vi "Heat2D_Solve X Direction.vi"(4 "F(t, x, y)":dbl[][][](array[numeric]), 5 "Coefficients":T2, 6 "step":i32, 7 "TriDia Cluster":T1, 8 "Boundary Condition":cluster{"type":T3, "Value":dbl[][]}[](array[cluster]) {"type" items=["Dirichlet", "Neumann"]}, 9 "U(n)":dbl[][](array[numeric]), 10 "Matr_RHS":dbl[][](array[numeric]), 11 "X RHS":dbl[][](array[numeric])) -> (1 "U(n+1/2)":dbl[][](array[numeric]), 3 "X RHS out":dbl[][](array[numeric]))   [LabVIEW 2020, in "NI_PDE.lvlib"]
uses:
  <vilib>/gmath/NI_PDE.lvlib
  <vilib>/gmath/pde.llb/Common/PDE_BC Type.ctl
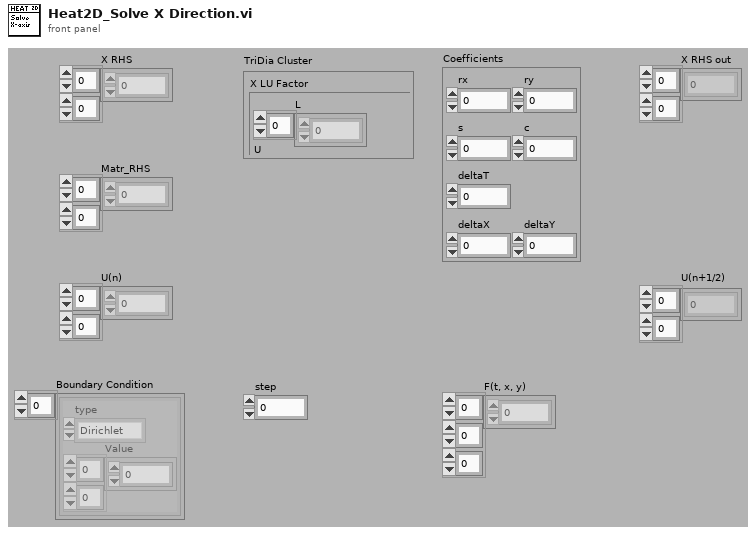
[diagram p1: front panel]
types:
  T1 = cluster{"X LU Factor":cluster{"L":dbl[], "U":cluster{"Diagonal":dbl[], "Super Diagonal":dbl[], "2nd Super Diagonal":dbl[]}, "Pivot":i32[]}, "Y LU Factor":cluster{"L":dbl[], "U":cluster{"Diagonal":dbl[], "Super Diagonal":dbl[], "2nd Super Diagonal":dbl[]}, "Pivot":i32[]}, "X Tridiagonal":cluster{"SubDiagonal":dbl[], "MainDiagonal":dbl[], "SuperDiagonal":dbl[]}, "Y Tridiagonal":cluster{"SubDiagonal":dbl[], "MainDiagonal":dbl[], "SuperDiagonal":dbl[]}}
  T2 = cluster{"rx":dbl, "ry":dbl, "s":dbl, "c":dbl, "deltaT":dbl, "deltaX":dbl, "deltaY":dbl}
  T3 = typedef "NI_PDE.lvlib/PDE_BC Type.ctl" = i32
  T4 = cluster{"L":dbl[], "U":cluster{"Diagonal":dbl[], "Super Diagonal":dbl[], "2nd Super Diagonal":dbl[]}, "Pivot":i32[]}
  T5 = cluster{"SubDiagonal":dbl[], "MainDiagonal":dbl[], "SuperDiagonal":dbl[]}
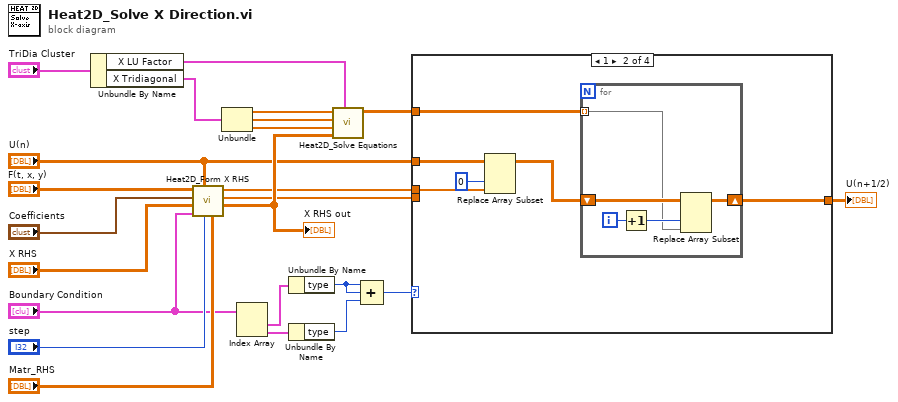
[diagram p0: block diagram]
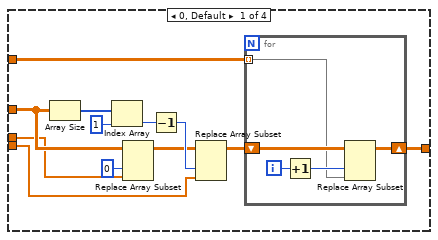
[diagram p2: hidden frame]
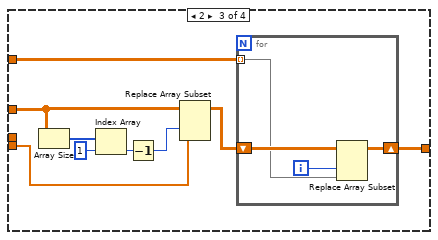
[diagram p3: hidden frame]
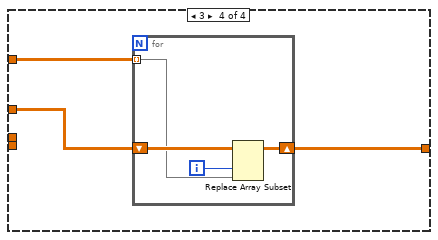
[diagram p4: hidden frame]
diagram:
  n1 = Unbundle By Name("TriDia Cluster") -> ("X LU Factor"=w10:T4, "X Tridiagonal"=w9:T5)
  n2 = call <vilib>:"Heat2D_Form X RHS.vi"("Matr_RHS"="Matr_RHS", "step"="step", "U(n)"="U(n)", "Boundary Condition"="Boundary Condition", "X RHS"="X RHS", "Coefficients"="Coefficients", "F(t, x, y)"="F(t, x, y)") -> ("X RHS out"=w13:dbl[][], "U(M)"=w1:dbl[], "U(0)"=w4:dbl[])  [unwired: 2 out]
  "X RHS out" <- w13
  n3 = Unbundle(w9) -> ("SubDiagonal"=w16:dbl[], "MainDiagonal"=w15:dbl[], "SuperDiagonal"=w14:dbl[])
  n4 = Index Array(array="Boundary Condition") -> (element #1=w20:cluster{"type":T3, "Value":dbl[][]}, element #2=w19:cluster{"type":T3, "Value":dbl[][]})  [unwired: 2 in]
  n5 = Unbundle By Name(w20) -> ("type"=w18:T3)
  n6 = Unbundle By Name(w19) -> ("type"=w17:T3)
  n7 = call <vilib>:"Heat2D_Solve Equations.vi"("LU Factor"=w10, "RHS"=w13, "SuperDiagonal"=w14, "MainDiagonal"=w15, "SubDiagonal"=w16) -> ("Solution Vector"=w6:dbl[][])  [unwired: 6 out]
  n8 = Compound Arithmetic op=ADD(w18, w18, w17) -> (w3:T3)
  n9 = case shown="1" w3 {
    tunnel: w6 -> [w26 w43 w53 w66]
    tunnel: [w25 w41 w52 w65] -> w2
    tunnel: w4 -> [w28 w45 _ _]
    tunnel: w1 -> [w24 _ w55 _]
    tunnel: "U(n)" -> [w29 w46 w56 w67]
    frame 0, Default {
      n10 = Array Size(array=w29) -> (size(s)=w31:i32[])
      n11 = Index Array(array=w31, index=1) -> (element=w32:i32)
      n12 = Replace Array Subset(array=w29, new element=w28, index (col)=0 ("index (row)")) -> (w30:dbl[][])  [unwired: 1 in]
      n13 = Decrement(x=w32) -> (x-1=w35:i32)
      n14 = Replace Array Subset(array=w30, new element=w24, index (col)=w35) -> (w27:dbl[][])  [unwired: 1 in]
      n15 = for {
        tunnel: w26 -> [w37] mode=indexing
        shift-right: [w36] -> w25
        shift-left: w27 -> [w40]
        i -> [w39]
        n16 = Increment(x=w39) -> (x+1=w38:i32)
        n17 = Replace Array Subset(array=w40, new element=w37, index (col)=w38) -> (w36:dbl[][])  [unwired: 1 in]
      }
    }
    frame 1 {
      n18 = Replace Array Subset(array=w46, new element=w45, index (col)=0 ("index (row)")) -> (w42:dbl[][])  [unwired: 1 in]
      n19 = for {
        tunnel: w43 -> [w48] mode=indexing
        shift-right: [w47] -> w41
        shift-left: w42 -> [w51]
        i -> [w50]
        n20 = Increment(x=w50) -> (x+1=w49:i32)
        n21 = Replace Array Subset(array=w51, new element=w48, index (col)=w49) -> (w47:dbl[][])  [unwired: 1 in]
      }
    }
    frame 2 {
      n22 = Array Size(array=w56) -> (size(s)=w59:i32[])
      n23 = Index Array(array=w59, index=1) -> (element=w60:i32)
      n24 = Decrement(x=w60) -> (x-1=w58:i32)
      n25 = Replace Array Subset(array=w56, new element=w55, index (col)=w58) -> (w54:dbl[][])  [unwired: 1 in]
      n26 = for {
        tunnel: w53 -> [w63] mode=indexing
        shift-right: [w62] -> w52
        shift-left: w54 -> [w64]
        i -> [w61]
        n27 = Replace Array Subset(array=w64, new element=w63, index (col)=w61) -> (w62:dbl[][])  [unwired: 1 in]
      }
    }
    frame 3 {
      n28 = for {
        tunnel: w66 -> [w70] mode=indexing
        shift-right: [w69] -> w65
        shift-left: w67 -> [w71]
        i -> [w68]
        n29 = Replace Array Subset(array=w71, new element=w70, index (col)=w68) -> (w69:dbl[][])  [unwired: 1 in]
      }
    }
  }
  "U(n+1/2)" <- w2
